vi "Chart & graph.vi"() -> ()   [LabVIEW 2012]
doc: "M. Ferrari Chart & Graph Functions"
panel:
  out "transposed array":dbl[][](array[numeric])
  out "Waveform \nGraph":cluster{"Xo":i32, "Dx":sgl, dbl[]}(graph) caption="Waveform Graph"
  out "clst vet":cluster{"vetx":dbl[], "vety":dbl[]}={"vetx"=[0.05866854037689562, 0.14184023240031918, 0.7442683626143671, 0.3494294931651645, 0.3836356278375954, 0.7348839856344198, 0.1539450093065724, 0.9654150415290764, 0.21734143685713048, 0.5622173281859761, 0.6162124214823783, 0.1664522163305322, 0.13357270779242425, 0.7573869007361198, 0.014148423405602628, 0.646305266764984, 0.2257604923756269, 0.307486380507489, 0.7646366160369646, 0.43061097848193164, 0.6521926314692204, 0.18421501620049652, 0.9771343651397116, 0.8053295370204466, 0.40287683614416414, 0.46924359801722826, 0.4584292584567804, 0.4830985877660581, 0.25799524008159547, 0.6066963876842288, 0.6395702455541402, 0.9992331136459148, 0.4317834511780174, 0.588295730374752, 0.425359564024411, 0.2586245440118351, 0.4664187036305427, 0.04504977258752163, 0.9940543951275798, 0.26865463690451014, 0.04510786195892624, 0.9560883509919212, 0.45216532465342674, 0.09259494335311214, 0.6530903377987971, 0.1316025875299882, 0.5420783119283707, 0.45659821097291453, 0.24295669024425326, 0.17129346045262372, 0.5455566170727997, 0.8350956088752046, 0.24048602999498803, 0.019960317887730117, 0.7723202339812217, 0.010690424235726415, 0.39647369871284166, 0.6683281012693525, 0.9353130639181463, 0.09041439619202185, 0.08946303218336737, 0.2949860412464915, 0.04926592690601739, 0.24734840233485644, 0.18976445473863124, 0.057782824683781486, 0.030700856306351554, 0.7888637202636988, 0.9813034848144941, 0.21498474739441775, 0.5387478200740241, 0.16183262783394836, 0.3202275290345382, 0.6452264688468958, 0.614351405076607, 0.06024446958334284, 0.9247499991340695, 0.23082800394664527, 0.2530374840553842, 0.09973742596786028, 0.4639765989889981, 0.3952908116565068, 0.9483062074644515, 0.33451324585897657, 0.15807892909647325, 0.8931079406674269, 0.7743800787238231, 0.010848687635037102, 0.8237657060364654, 0.2920527400594597, 0.3199134107691144, 0.1459267962252515, 0.7986338760439046, 0.5591419416105365, 0.8971398295095757, 0.5089051434358309, 0.2419446906169207, 0.9737748674567568, 0.7477415993586707, 0.24338965732332163], "vety"=[0.0, 3.0, 6.0, 9.0, 12.0, 15.0, 18.0, 21.0, 24.0, 27.0, 30.0, 33.0, 36.0, 39.0, 42.0, 45.0, 48.0, 51.0, 54.0, 57.0, 60.0, 63.0, 66.0, 69.0, 72.0, 75.0, 78.0, 81.0, 84.0, 87.0, 90.0, 93.0, 96.0, 99.0, 102.0, 105.0, 108.0, 111.0, 114.0, 117.0, 120.0, 123.0, 126.0, 129.0, 132.0, 135.0, 138.0, 141.0, 144.0, 147.0, 150.0, 153.0, 156.0, 159.0, 162.0, 165.0, 168.0, 171.0, 174.0, 177.0, 180.0, 183.0, 186.0, 189.0, 192.0, 195.0, 198.0, 201.0, 204.0, 207.0, 210.0, 213.0, 216.0, 219.0, 222.0, 225.0, 228.0, 231.0, 234.0, 237.0, 240.0, 243.0, 246.0, 249.0, 252.0, 255.0, 258.0, 261.0, 264.0, 267.0, 270.0, 273.0, 276.0, 279.0, 282.0, 285.0, 288.0, 291.0, 294.0, 297.0]} {"vety" format="%.2f"; "vetx" format="%.2f"}
  in  "N° points":i32=100
  out "XY sgraph":cluster{dbl[], i32[]}(graph)
  out "matr":dbl[][](array[numeric]) format="%.2f"
  in  "Delay":u32
  in  "N° xpoints":i32=10
  in  "Dx":sgl=1.0 format="%.2f"
  in  "Xo":i32
  out "w mgraph":cluster{"Xo":i32, "Dx":sgl, dbl[]}[](graph)
  in  "Delay":u32
  in  "N° sample":i32=10
  in  "Dx":sgl=1.0 format="%.2f"
  in  "Xo":i32
  in  "Tsample":u32=500
  in  "stop 1":bool
  out "w mchart":dbl[][](graph)
  in  "Tsample":u32=500
  in  "enabl":bool
  out "w chart":dbl(graph)
  # "WAVEFORM CHART  single plot"
  # "[ms]"
  # "WAVEFORM CHART  multiplot"
  # "[ms]"
  # "Tramite ' Advanced' sono possibili\ntre distinte modalità di rappresentazione\n(update mode) :\n- strip chart -\n- scope chart -\n- sweep chart -"
  # "WAVEFORM GRAPH single plot"
  # "WAVEFORM GRAPH multiplot"
  # "XY GRAPH single plot"
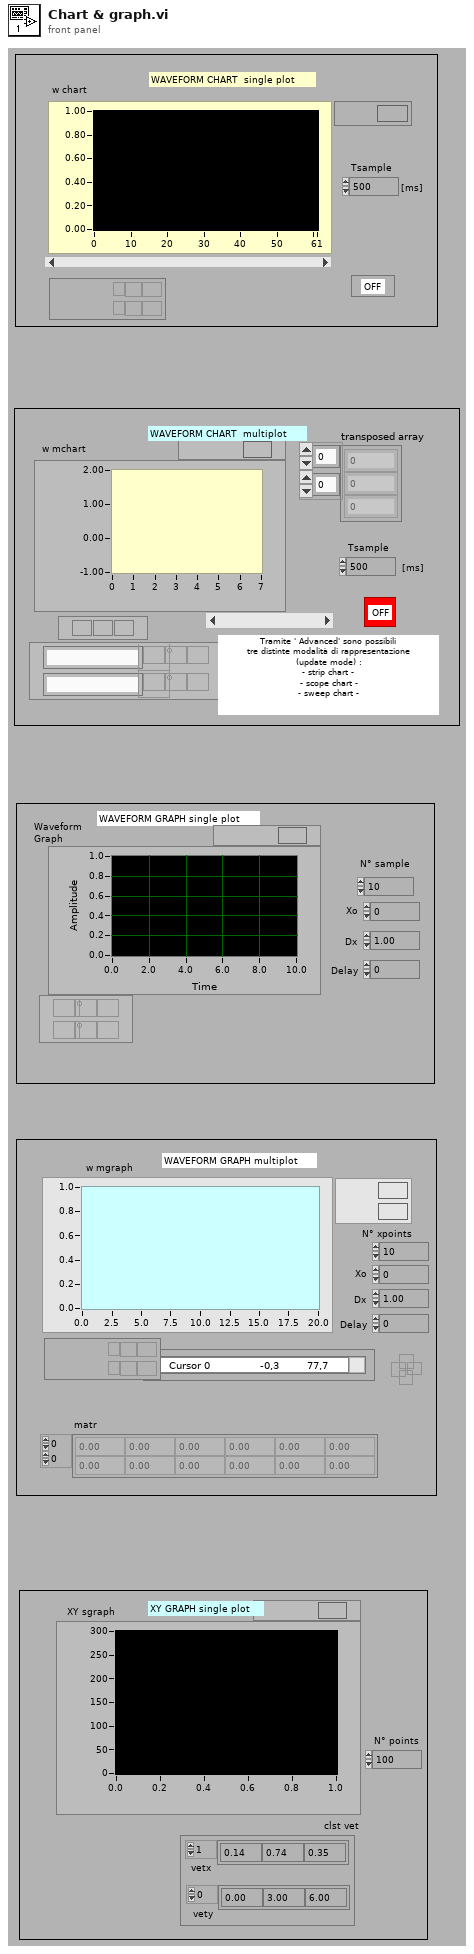
[diagram p1: front panel]
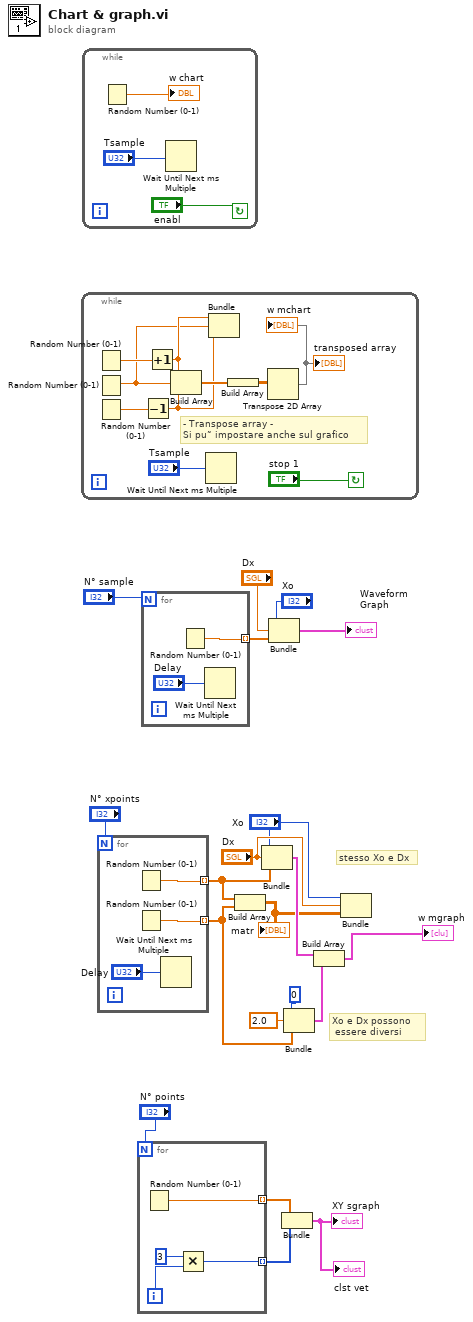
[diagram p0: block diagram]
diagram:
  # "Xo e Dx possono\n essere diversi"
  # "stesso Xo e Dx"
  n1 = while {
    stop <- "stop 1" continue-if-true
    # "- Transpose array -\nSi pu˜ impostare anche sul grafico"
    n2 = Random Number (0-1)() -> (number: 0 to 1=w30:dbl)
    n3 = Random Number (0-1)() -> (number: 0 to 1=w24:dbl)
    n4 = Random Number (0-1)() -> (number: 0 to 1=w29:dbl)
    n5 = Decrement(x=w29) -> (x-1=w23:dbl)
    n6 = Increment(x=w30) -> (x+1=w25:dbl)
    n7 = Build Array(w25, w24, w23) -> (w27:dbl[])
    n8 = Wait Until Next ms Multiple(millisecond multiple="Tsample") -> ()  [unwired: 1 out]
    n9 = Bundle(w25, "number: 0 to 1"=w24, w23) -> ()  [unwired: 1 in, 1 out]
    n10 = Build Array(w27) -> (w26:dbl[][])
    n11 = Transpose 2D Array(2D array=w26) -> (transposed array=→"w mchart" →"transposed array":dbl[][])
  }
  n12 = while {
    stop <- "enabl" continue-if-true
    n13 = Random Number (0-1)() -> (number: 0 to 1=→"w chart":dbl)
    n14 = Wait Until Next ms Multiple(millisecond multiple="Tsample") -> ()  [unwired: 1 out]
  }
  n15 = for {
    N: "N° xpoints" -> [_]
    tunnel: [w36] -> w8 mode=indexing
    tunnel: [w34] -> w10 mode=indexing
    n16 = Random Number (0-1)() -> (number: 0 to 1=w36:dbl)
    n17 = Random Number (0-1)() -> (number: 0 to 1=w34:dbl)
    n18 = Wait Until Next ms Multiple(millisecond multiple="Delay") -> ()  [unwired: 1 out]
  }
  n19 = for {
    N: "N° points" -> [_]
    tunnel: [w40] -> w5 mode=indexing
    tunnel: [w37] -> w3 mode=indexing
    i -> [w39]
    n20 = Random Number (0-1)() -> (number: 0 to 1=w40:dbl)
    n21 = Multiply(x=3, y=w39) -> (x*y=w37:i32)
  }
  n22 = for {
    N: "N° sample" -> [_]
    tunnel: [w41] -> w17 mode=indexing
    n23 = Random Number (0-1)() -> (number: 0 to 1=w41:dbl)
    n24 = Wait Until Next ms Multiple(millisecond multiple="Delay") -> ()  [unwired: 1 out]
  }
  n25 = Build Array(w8, w10) -> (w9:dbl[][])
  "matr" <- w9
  n26 = Bundle("Xo"="Xo", "Dx"="Dx", w8) -> (w12:cluster{"Xo":i32, "Dx":sgl, dbl[]})  [unwired: 1 in]
  n27 = Bundle("Xo"="Xo", "Dx"="Dx", w17) -> (→"Waveform \nGraph":cluster{"Xo":i32, "Dx":sgl, dbl[]})  [unwired: 1 in]
  n28 = Bundle(w5, w3) -> (→"XY sgraph" →"clst vet":cluster{dbl[], i32[]})  [unwired: 1 in]
  n29 = Bundle(0, sgl 2.0, w10) -> (w11:cluster{i32, sgl, dbl[]})  [unwired: 1 in]
  n30 = Build Array(w12, w11) -> (→"w mgraph":cluster{"Xo":i32, "Dx":sgl, dbl[]}[])
  n31 = Bundle("Xo"="Xo", "Dx"="Dx", w9) -> ()  [unwired: 1 in, 1 out]
